vi "Sending Waveforms to Origin.vi"() -> ()   [LabVIEW 2020]
uses:
  Instance           1 35Saved   Sending Waveforms to Origin .vi
  Instance           2 35Saved   Sending Waveforms to Origin .vi
panel:
  out "error IO":errorcluster
  out "Origin file path":path
  in  "stop":bool
  out "Waveform Chart":dynamicdata(graph)
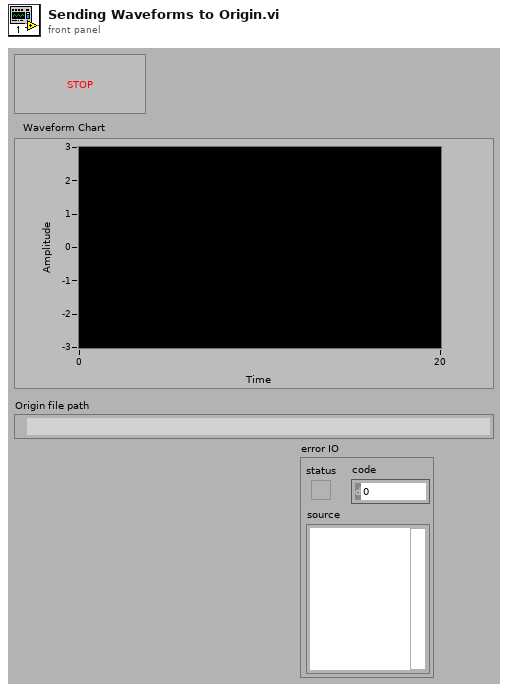
[diagram p1: front panel]
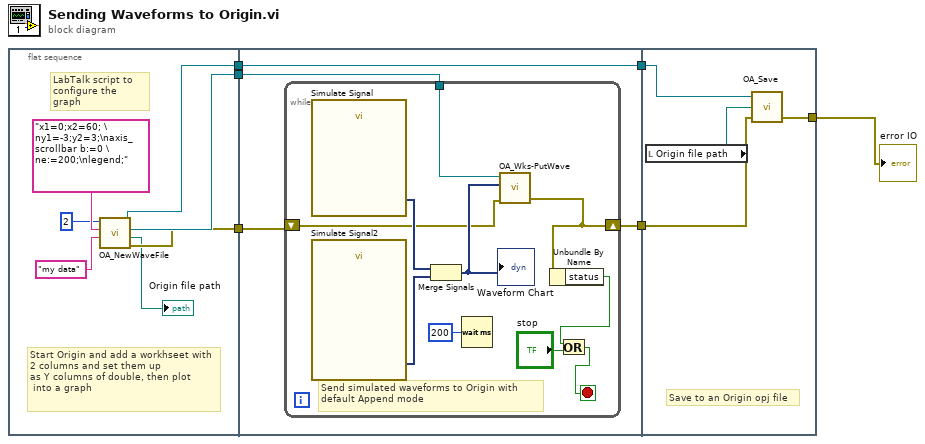
[diagram p0: block diagram]
diagram:
  n1 = flat-sequence {
    tunnel: [w13] -> w6
    tunnel: [w12] -> w4
    tunnel: [w11] -> w3
    tunnel: w6 -> [w17]
    tunnel: [w16] -> w5
    tunnel: w4 -> [w16]
    tunnel: w3 -> [w15]
    tunnel: [w14] -> w2
    tunnel: w5 -> [w31]
    tunnel: w2 -> [w29]
    tunnel: [w28] -> w1
    frame #0 {
      # "LabTalk script to\nconfigure the graph"
      # "Start Origin and add a workhseet with\n2 columns and set them up\nas Y columns of double, then plot\n into a graph"
      n2 = call "OA_NewWaveFile.vi"("Origin file name"="my data" ("Origin filename"), "graph script"="x1=0;x2=60; \ny1=-3;y2=3;\naxis_scrollbar b:=0 \ne:=200;\nlegend;", "number of columns"=2) -> ("error out"=w11:errorcluster, "path out"=→"Origin file path":path, "Origin.Worksheet"=w13:refnum<k7>, "Origin.IOApplication"=w12:refnum<k7>)  [unwired: 5 in]
    }
    frame #1 {
      n3 = while {
        tunnel: w17 -> [w24]
        shift-right: [w18] -> w14
        shift-left: w15 -> [w22]
        stop <- w20 stop-if-true
        # "Send simulated waveforms to Origin with \ndefault Append mode"
        n4 = call "Simulate Signal"() -> ("Sine with Uniform Noise"=w27:dynamicdata)  [unwired: 14 in, 1 out]
        n5 = call "Simulate Signal2"() -> ("Square with Uniform Noise"=w26:dynamicdata)  [unwired: 14 in, 1 out]
        n6 = Merge Signals(w27, w26) -> (w25:dynamicdata)
        "Waveform Chart" <- w25
        n7 = Wait (ms)(milliseconds to wait=u32 200) -> ()  [unwired: 1 out]
        n8 = call "OA_Wks-PutWave.vi"("Origin.Worksheet"=w24, "Dynamic Data"=w25, "error in (no error)"=w22) -> ("error IO"=w18:errorcluster)  [unwired: 3 in, 1 out]
        n9 = Unbundle By Name(w18) -> ("status"=w19:bool)
        n10 = Or(x=w19, y="stop") -> (x .or. y?=w20:bool)
      }
    }
    frame #2 {
      # "Save to an Origin opj file"
      n11 = local read "Origin file path"() -> (w30:path)
      n12 = call "OA_Save.vi"("Error IO"=w29, "Path"=w30, "Origin.IOApplication"=w31) -> ("Error IO Out"=w28:errorcluster)  [unwired: 2 out]
    }
  }
  "error IO" <- w1
